vi "dot frame and fill placement.vi"(6 "Color":u32(colorbox)=16711680, 8 "Drawing Mode (Frame)":u32(ring) items=["Frame", "Fill"], 9 "y coordinate":sgl, 10 "x coordinate":sgl, 11 "Image":T1) -> (3 "Image Out":T1)   [LabVIEW 2018]
uses:
  <vilib>/vision/Image Controls.llb/IMAQ Image.ctl
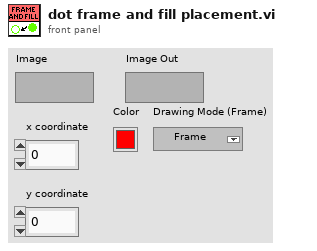
[diagram p1: front panel]
types:
  T1 = typedef "IMAQ Image.ctl" = refnum<image>
  T2 = cluster{"Left":i32, "Top":i32, "Right":i32, "Bottom":i32}
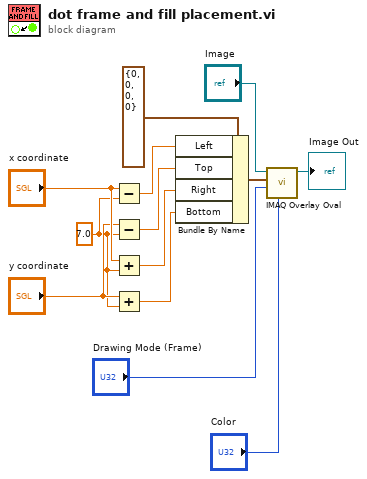
[diagram p0: block diagram]
diagram:
  w6 = sgl 7.0 ("y")
  n1 = Subtract(x="x coordinate", y=w6) -> (x-y=w5:sgl)
  n2 = Subtract(x="y coordinate", y=w6) -> (x-y=w2:sgl)
  n3 = Add(x="x coordinate", y=w6) -> (x+y=w4:sgl)
  n4 = Add(x="y coordinate", y=w6) -> (x+y=w3:sgl)
  n5 = Bundle By Name(cluster=T2 {"Left"=0, "Top"=0, "Right"=0, "Bottom"=0} ("Bounding Rectangle"), "Left"=w5, "Top"=w2, "Right"=w4, "Bottom"=w3) -> (w12:T2)
  n6 = call "IMAQ Overlay Oval"("Color"="Color", "Drawing Mode (Frame)"="Drawing Mode (Frame)", "Bounding Rectangle"=w12, "Image"="Image") -> ("Image Out"=→"Image Out":T1)  [unwired: 6 in, 1 out]
